vi "Read data type.vi"(8 "error in (no error)":errorcluster, 11 "DSFChannel in":refnum<class "DSFChannel.lvclass">) -> (0 "error out":errorcluster, 2 "data type":T1, 3 "DSFChannel out":refnum<class "DSFChannel.lvclass">)   [LabVIEW 2017, in "DSFChannel.lvclass"]
uses:
  DSFChannel.lvclass
  dsf channel data type.ctl
  DSFChannel.lvclass/DSFChannel.ctl
  5675bfa6-582b-4280-b3d1-3aa885c4c239.vi
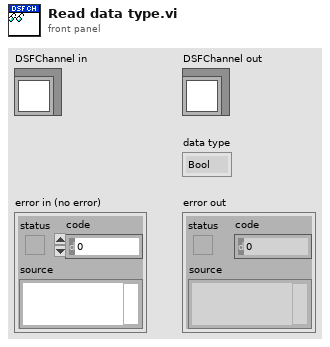
[diagram p1: front panel]
types:
  T1 = typedef "DSFChannel.lvclass/dsf channel data type.ctl" = enum32{"Bool", "SGL", "DBL", "I8", "I16", "I32", "I64", "U8", "U16", "U32", "U64"}
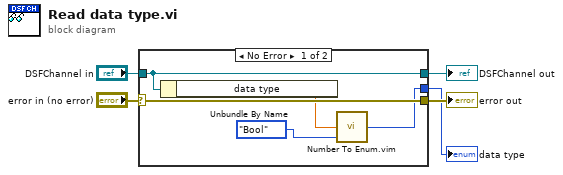
[diagram p0: block diagram]
diagram:
  n1 = case shown="No Error" "error in (no error)" {
    selector: "error in (no error)" -> [w10 w11]
    tunnel: [w10 w11] -> w4
    tunnel: [w9 w12] -> w2
    tunnel: "DSFChannel in" -> [w9 w12]
    tunnel: [w6 _] -> w1
    frame No Error {
      n2 = Unbundle By Name(w9) -> ("data type"=w8:dbl)
      n3 = call "Number To Enum.vim"("number"=w8, "enum type"=dsf_channel_data_type."Bool" ("data type")) -> ("number as enum"=w6:T1)
    }
    frame Error {
    }
  }
  "error out" <- w4
  "DSFChannel out" <- w2
  "data type" <- w1
